vi "Freq Filter(SubVI).vi"(6 "Lower Freq":dbl, 9 "Upper Freq":dbl, 10 "amplitude":dbl, 11 "Frequency":dbl) -> (2 "Tunnel?":bool, 3 "Cluster":cluster{dbl, "y":dbl})   [LabVIEW 2017]
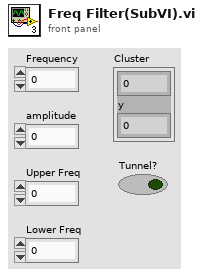
[diagram p1: front panel]
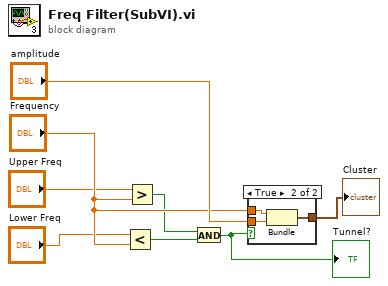
[diagram p0: block diagram]
diagram:
  n1 = Less?(x="Lower Freq", y="Frequency") -> (x < y?=w3:bool)
  n2 = Greater?(x="Upper Freq", y="Frequency") -> (0:w2:bool)
  n3 = And(x=w2, y=w3) -> (x .and. y?=w8:bool)
  "Tunnel?" <- w8
  n4 = case shown="True" w8 {
    tunnel: "Frequency" -> [_ w11]
    tunnel: "amplitude" -> [_ w10]
    tunnel: [_ w9] -> w1
    frame False {
    }
    frame True {
      n5 = Bundle("Frequency"=w11, "amplitude"=w10) -> (w9:cluster{"Frequency":dbl, "amplitude":dbl})  [unwired: 1 in]
    }
  }
  "Cluster" <- w1
